vi "Project-overflow.vi"() -> ()   [LabVIEW 2016]
uses:
  <vilib>/DAQmx/read.llb/DAQmx Read (Digital Bool 1Line 1Point).vi
  <vilib>/DAQmx/write.llb/DAQmx Write (Digital Bool 1Line 1Point).vi
  <vilib>/DAQmx/create/channels.llb/DAQmx Create Channel (DO-Digital Output).vi
  <vilib>/DAQmx/create/channels.llb/DAQmx Create Channel (DI-Digital Input).vi
  <vilib>/DAQmx/miscellaneous.llb/DAQmx Fill In Error Info.vi
  <vilib>/ptbypt/NI_PtbyPt.lvlib
panel:
  out "Use R3":bool
  out "Register Bit 3":bool
  out "Laser Sensor":bool
  out "Use R2":bool
  out "Use R1":bool
  out "Register Bit 1":bool
  out "Register Bit 2":bool
  out "Output Queue Counter":dbl
  out "Rejection Pusher":bool
  out "Metal Sensor 2":bool
  out "Inductive Sensor":bool
  out "Complete or not":bool
  out "Plastic In Queue":dbl
  out "Hopper":bool
  out "Pusher":bool=TRUE
  out "Plastic or not":bool
  out "Belt 2":bool=TRUE
  out "Belt 1":bool=TRUE
  out "Stoped":bool=TRUE
  out "Started":bool=TRUE
  in  "PAUSE":bool
  in  "OFF":bool
  in  "ON":bool
  out "Rejected Pieces":dbl
  out "Completed Pieces":dbl
  out "Don't Push?":bool
  in  "Emergency Stop":bool
  out "Is there anything there?":bool
  # "Main Control"
  # "Sorting Station"
  # "QA Sorting Station"
  # "QA Sorting Register Value"
  # "Result Counter"
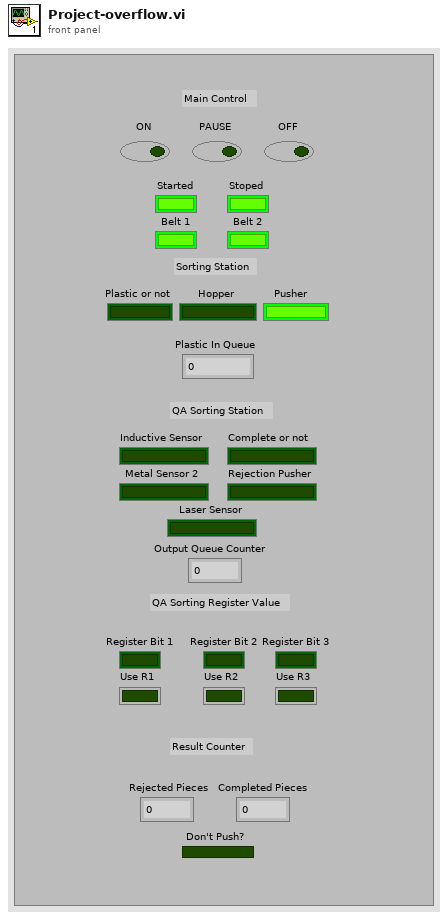
[diagram p1: front panel]
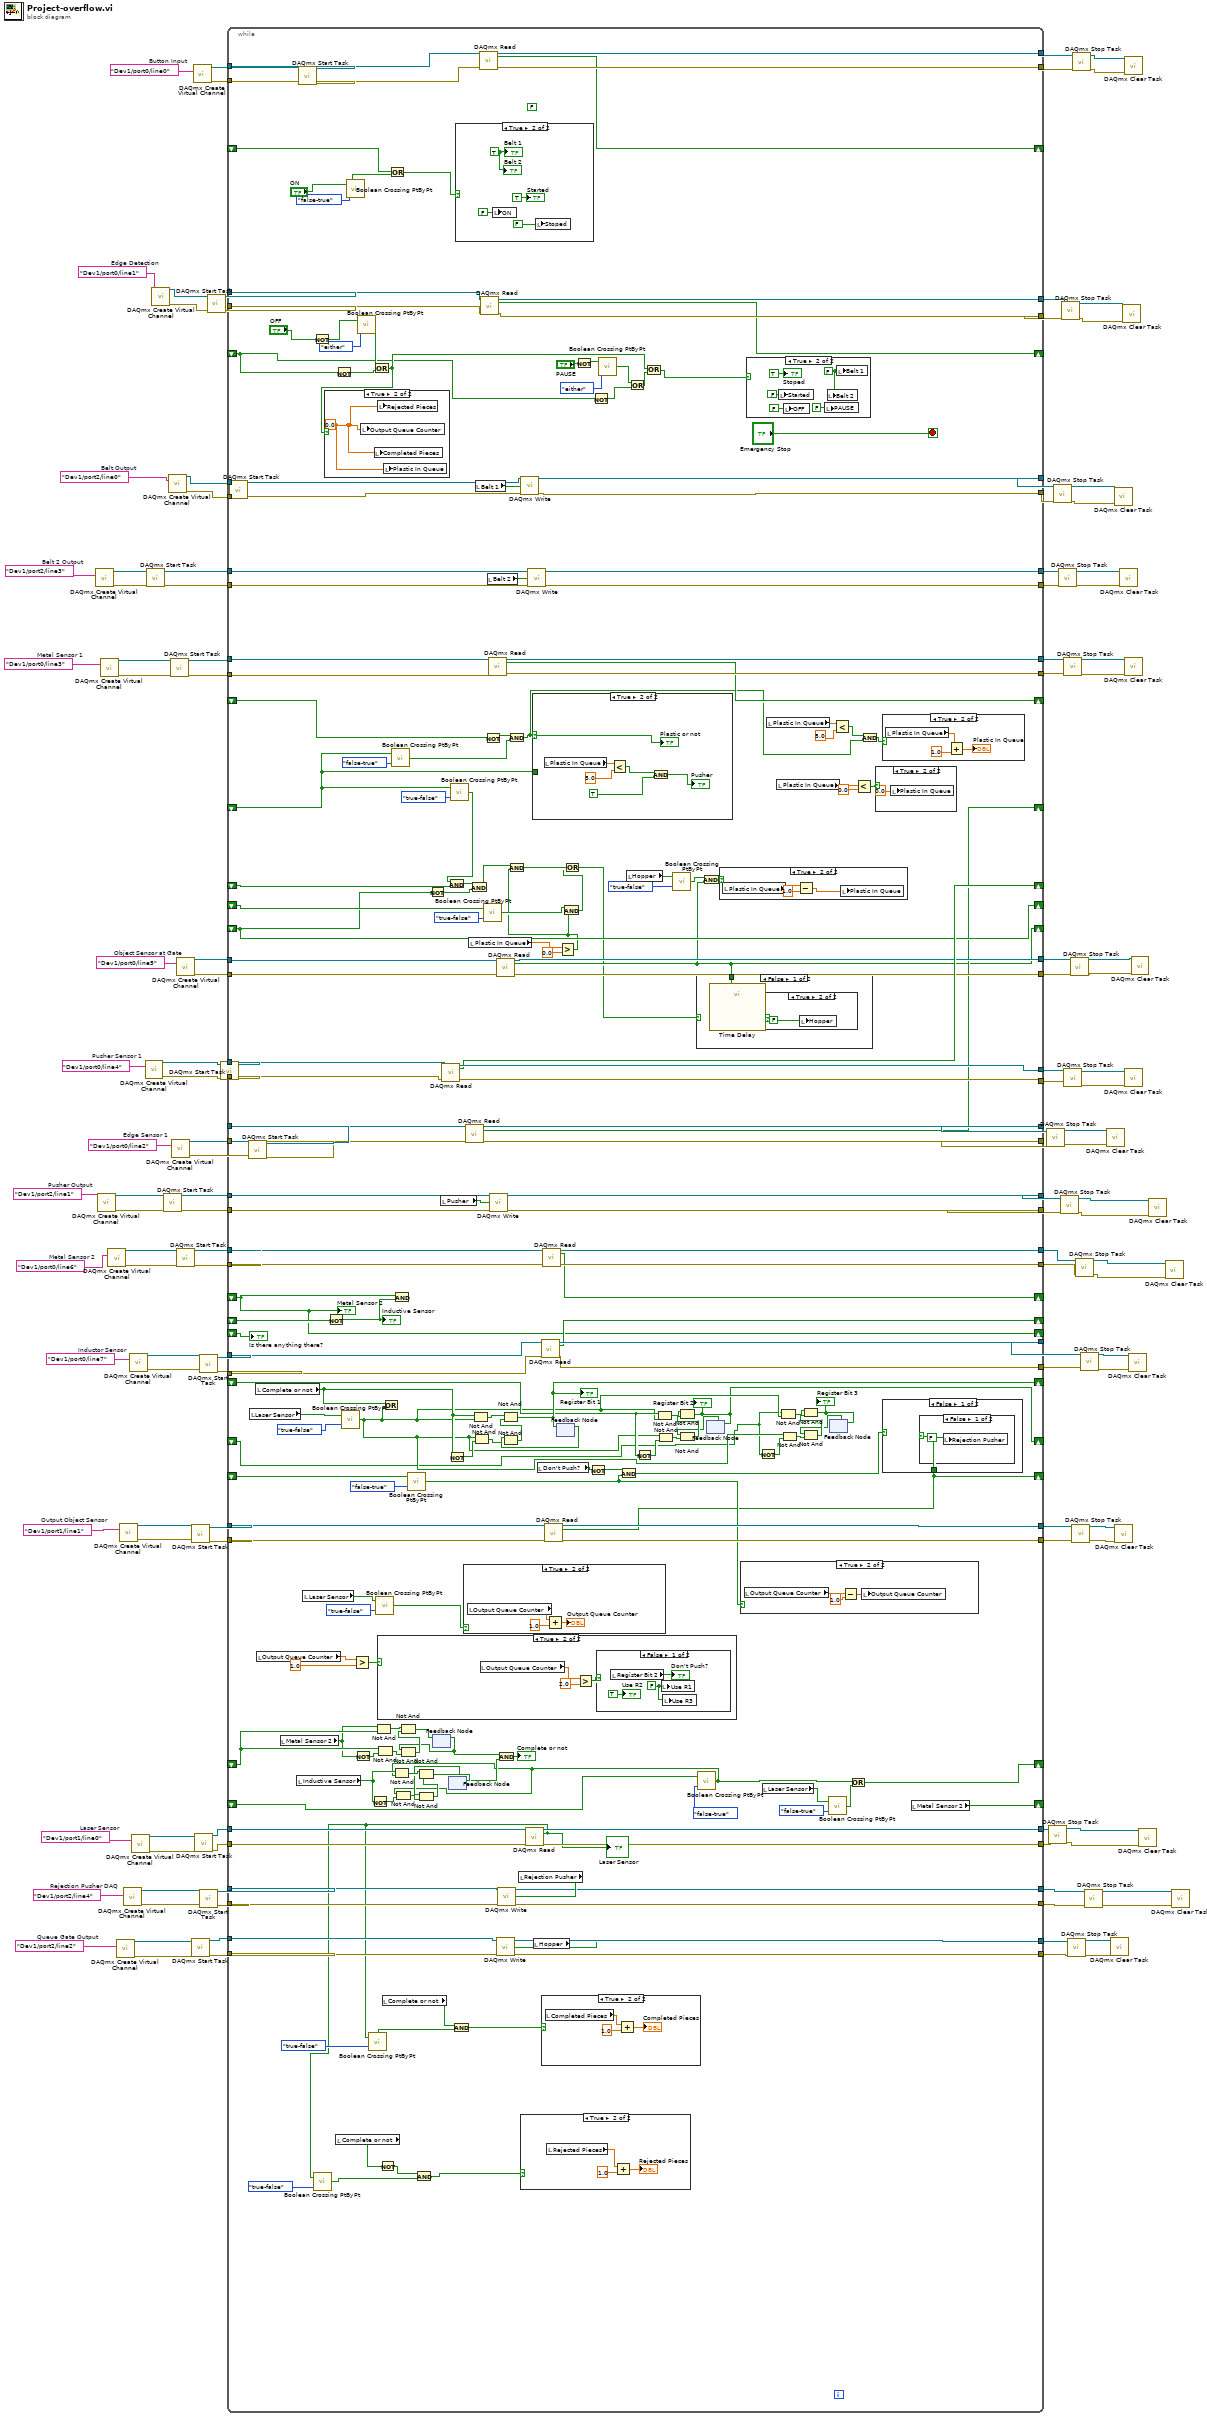
[diagram p0: block diagram]
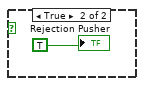
[diagram p3: hidden frame]
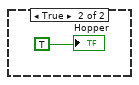
[diagram p5: hidden frame]
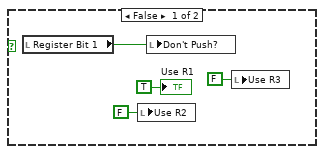
[diagram p12: hidden frame]
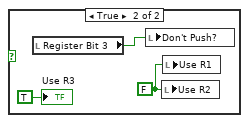
[diagram p13: hidden frame]
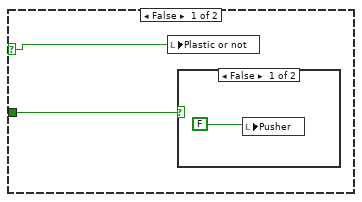
[diagram p16: hidden frame]
diagram:
  w5 = tag "Dev1/port0/line5"  # Object Sensor at Gate
  w12 = tag "Dev1/port1/line0"  # Laser Sensor
  w25 = tag "Dev1/port0/line7"  # Inductor Sensor
  w28 = tag "Dev1/port1/line1"  # Output Object Sensor
  w43 = tag "Dev1/port0/line6"  # Metal Sensor 2
  w46 = tag "Dev1/port2/line4"  # Rejection Pusher DAQ
  w57 = tag "Dev1/port2/line2"  # Queue Gate Output
  w64 = tag "Dev1/port2/line3"  # Belt 2 Output
  w75 = tag "Dev1/port0/line4"  # Pusher Sensor 1
  w84 = tag "Dev1/port0/line2"  # Edge Sensor 1
  w89 = tag "Dev1/port2/line1"  # Pusher Output
  w90 = tag "Dev1/port0/line1"  # Edge Detection
  w91 = tag "Dev1/port0/line0"  # Button Input
  w92 = tag "Dev1/port0/line3"  # Metal Sensor 1
  w93 = tag "Dev1/port2/line0"  # Belt Output
  n1 = call-poly <vilib>:"DAQmx Create Virtual Channel.vi"("lines"=w64) -> ("task out"=w66:refnum<k21>, "error out"=w65:errorcluster)  [unwired: 13 in]
  n2 = call-poly <vilib>:"DAQmx Create Virtual Channel.vi"("lines"=w89) -> ("task out"=w101:refnum<k21>, "error out"=w100:errorcluster)  [unwired: 13 in]
  n3 = call-poly <vilib>:"DAQmx Create Virtual Channel.vi"("lines"=w92) -> ("task out"=w109:refnum<k21>, "error out"=w108:errorcluster)  [unwired: 13 in]
  n4 = call-poly <vilib>:"DAQmx Create Virtual Channel.vi"("lines"=w43) -> ("task out"=w45:refnum<k21>, "error out"=w44:errorcluster)  [unwired: 13 in]
  n5 = call-poly <vilib>:"DAQmx Create Virtual Channel.vi"("lines"=w57) -> ("task out"=w59:refnum<k21>, "error out"=w58:errorcluster)  [unwired: 13 in]
  n6 = call-poly <vilib>:"DAQmx Create Virtual Channel.vi"("lines"=w28) -> ("task out"=w30:refnum<k21>, "error out"=w29:errorcluster)  [unwired: 13 in]
  n7 = call-poly <vilib>:"DAQmx Create Virtual Channel.vi"("lines"=w46) -> ("task out"=w48:refnum<k21>, "error out"=w47:errorcluster)  [unwired: 13 in]
  n8 = call-poly <vilib>:"DAQmx Create Virtual Channel.vi"("lines"=w25) -> ("task out"=w27:refnum<k21>, "error out"=w26:errorcluster)  [unwired: 13 in]
  n9 = call-poly <vilib>:"DAQmx Create Virtual Channel.vi"("lines"=w12) -> ("task out"=w14:refnum<k21>, "error out"=w13:errorcluster)  [unwired: 13 in]
  n10 = call-poly <vilib>:"DAQmx Create Virtual Channel.vi"("lines"=w75) -> ("task out"=w77:refnum<k21>, "error out"=w76:errorcluster)  [unwired: 13 in]
  n11 = call <vilib>:"DAQmx Start Task.vi"("task/channels in"=w66, "error in"=w65) -> ("task out"=w63:refnum<k21>, "error out"=w62:errorcluster)  [unwired: 12 in]
  n12 = call-poly <vilib>:"DAQmx Create Virtual Channel.vi"("lines"=w90) -> ("task out"=w125:refnum<k21>, "error out"=w124:errorcluster)  [unwired: 13 in]
  n13 = call <vilib>:"DAQmx Start Task.vi"("task/channels in"=w101, "error in"=w100) -> ("task out"=w95:refnum<k21>, "error out"=w94:errorcluster)  [unwired: 12 in]
  n14 = call-poly <vilib>:"DAQmx Create Virtual Channel.vi"("lines"=w93) -> ("task out"=w113:refnum<k21>, "error out"=w112:errorcluster)  [unwired: 13 in]
  n15 = call <vilib>:"DAQmx Start Task.vi"("task/channels in"=w109, "error in"=w108) -> ("task out"=w107:refnum<k21>, "error out"=w106:errorcluster)  [unwired: 12 in]
  n16 = call-poly <vilib>:"DAQmx Create Virtual Channel.vi"("lines"=w84) -> ("task out"=w86:refnum<k21>, "error out"=w85:errorcluster)  [unwired: 13 in]
  n17 = call <vilib>:"DAQmx Start Task.vi"("task/channels in"=w45, "error in"=w44) -> ("task out"=w40:refnum<k21>, "error out"=w39:errorcluster)  [unwired: 12 in]
  n18 = call-poly <vilib>:"DAQmx Create Virtual Channel.vi"("lines"=w5) -> ("task out"=w4:refnum<k21>, "error out"=w3:errorcluster)  [unwired: 13 in]
  n19 = call <vilib>:"DAQmx Start Task.vi"("task/channels in"=w30, "error in"=w29) -> ("task out"=w24:refnum<k21>, "error out"=w23:errorcluster)  [unwired: 12 in]
  n20 = call <vilib>:"DAQmx Start Task.vi"("task/channels in"=w59, "error in"=w58) -> ("task out"=w56:refnum<k21>, "error out"=w55:errorcluster)  [unwired: 12 in]
  n21 = call-poly <vilib>:"DAQmx Create Virtual Channel.vi"("lines"=w91) -> ("task out"=w133:refnum<k21>, "error out"=w132:errorcluster)  [unwired: 13 in]
  n22 = call <vilib>:"DAQmx Start Task.vi"("task/channels in"=w14, "error in"=w13) -> ("task out"=w11:refnum<k21>, "error out"=w8:errorcluster)  [unwired: 12 in]
  n23 = call <vilib>:"DAQmx Start Task.vi"("task/channels in"=w27, "error in"=w26) -> ("task out"=w22:refnum<k21>, "error out"=w21:errorcluster)  [unwired: 12 in]
  n24 = call <vilib>:"DAQmx Start Task.vi"("task/channels in"=w48, "error in"=w47) -> ("task out"=w38:refnum<k21>, "error out"=w37:errorcluster)  [unwired: 12 in]
  n25 = call <vilib>:"DAQmx Start Task.vi"("task/channels in"=w125, "error in"=w124) -> ("task out"=w122:refnum<k21>, "error out"=w123:errorcluster)  [unwired: 12 in]
  n26 = call <vilib>:"DAQmx Start Task.vi"("task/channels in"=w77, "error in"=w76) -> ("task out"=w74:refnum<k21>, "error out"=w73:errorcluster)  [unwired: 12 in]
  n27 = call <vilib>:"DAQmx Start Task.vi"("task/channels in"=w113, "error in"=w112) -> ("task out"=w111:refnum<k21>, "error out"=w110:errorcluster)  [unwired: 12 in]
  n28 = call <vilib>:"DAQmx Start Task.vi"("task/channels in"=w86, "error in"=w85) -> ("task out"=w83:refnum<k21>, "error out"=w82:errorcluster)  [unwired: 12 in]
  n29 = call <vilib>:"DAQmx Start Task.vi"("task/channels in"=w133, "error in"=w132) -> ("task out"=w131:refnum<k21>, "error out"=w130:errorcluster)  [unwired: 12 in]
  n30 = while {
    tunnel: w131 -> [w334]
    tunnel: w130 -> [w333]
    tunnel: [w332] -> w129
    tunnel: [w331] -> w128
    shift-right: [w329] -> _
    shift-left: _ -> [w263]
    tunnel: w123 -> [w328]
    tunnel: w122 -> [w327]
    tunnel: [w326] -> w121
    tunnel: [w325] -> w118
    shift-right: [w324] -> _
    shift-left: _ -> [w203]
    tunnel: [w323] -> w115
    tunnel: [w320] -> w114
    tunnel: w111 -> [w322]
    tunnel: w110 -> [w321]
    tunnel: w107 -> [w318]
    tunnel: w106 -> [w317]
    tunnel: [w316] -> w103
    tunnel: [w315] -> w102
    shift-right: [w178] -> _
    shift-left: _ -> [w177]
    tunnel: [w313] -> w97
    tunnel: [w312] -> w96
    tunnel: w95 -> [w311]
    tunnel: w94 -> [w310]
    tunnel: w83 -> [w309]
    tunnel: w82 -> [w308]
    tunnel: [w307] -> w81
    tunnel: [w306] -> w80
    shift-right: [w180] -> _
    shift-left: _ -> [w173]
    tunnel: w74 -> [w304]
    tunnel: w73 -> [w303]
    tunnel: [w302] -> w72
    tunnel: [w301] -> w71
    tunnel: [w298] -> w68
    tunnel: [w297] -> w67
    tunnel: w63 -> [w296]
    tunnel: w62 -> [w295]
    tunnel: w56 -> [w294]
    tunnel: w55 -> [w293]
    tunnel: [w292] -> w54
    tunnel: [w291] -> w53
    shift-right: [w289] -> _
    shift-left: _ -> [w288]
    tunnel: [w284] -> w42
    tunnel: [w283] -> w41
    tunnel: w40 -> [w282]
    tunnel: w39 -> [w281]
    tunnel: w38 -> [w280]
    tunnel: w37 -> [w279]
    tunnel: [w278] -> w36
    tunnel: [w277] -> w35
    shift-right: [w276] -> _
    shift-left: _ -> [w230]
    tunnel: w24 -> [w275]
    tunnel: w23 -> [w274]
    tunnel: w22 -> [w273]
    tunnel: w21 -> [w272]
    tunnel: [w271] -> w20
    tunnel: [w270] -> w19
    tunnel: [w269] -> w18
    tunnel: [w268] -> w17
    shift-right: [w181] -> _
    shift-left: _ -> [w251]
    shift-right: [w267] -> _
    shift-left: _ -> [w266]
    shift-right: [w230] -> _
    shift-left: _ -> [w253]
    tunnel: w11 -> [w249]
    tunnel: [w248] -> w10
    tunnel: [w247] -> w9
    tunnel: w8 -> [w246]
    shift-right: [w232] -> _
    shift-left: _ -> [w231]
    tunnel: w4 -> [w202]
    tunnel: w3 -> [w201]
    tunnel: [w200] -> w2
    tunnel: [w199] -> w1
    shift-right: [w175] -> _
    shift-left: _ -> [w194]
    shift-right: [w194] -> _
    shift-left: _ -> [w197]
    shift-right: [w154] -> _
    shift-left: _ -> [w166]
    shift-right: [w137] -> _
    shift-left: _ -> [w136]
    shift-right: [w135] -> _
    shift-left: _ -> [w134]
    stop <- "Emergency Stop" stop-if-true
    (unwired) FALSE ("Boolean")
    n31 = local read "Laser Sensor"() -> (w254:bool)
    n32 = local read "Complete or not"() -> (w229:bool)
    n33 = local read "Output Queue Counter"() -> (w239:dbl)
    n34 = local read "Metal Sensor 2"() -> (w165:bool)
    n35 = local read "Inductive Sensor"() -> (w159:bool)
    n36 = local read "Laser Sensor"() -> (w243:bool)
    n37 = Not(x="OFF") -> (.not. x?=w225:bool)
    n38 = Not(x=w266) -> (.not. x?=w261:bool)
    "Inductive Sensor" <- w261
    n39 = Not(x=w203) -> (.not. x?=w262:bool)
    n40 = local read "Complete or not"() -> (w212:bool)
    n41 = call <vilib>:"Boolean Crossing PtByPt.vi"("direction"=enum16{"either", "false-true", "true-false"}."true-false", "input"=w254) -> ("crossing"=w144:bool)  [unwired: 1 in]
    n42 = call <vilib>:"Boolean Crossing PtByPt.vi"("direction"=enum16{"either", "false-true", "true-false"}."false-true", "input"="ON") -> ("crossing"=w228:bool)  [unwired: 1 in]
    n43 = Greater?(x=w239, y=1.0) -> (0:w238:bool)
    n44 = Not(x=w165) -> (.not. x?=w169:bool)
    n45 = call <vilib>:"Boolean Crossing PtByPt.vi"("direction"=enum16{"either", "false-true", "true-false"}."either", "input"=w225) -> ("crossing"=w226:bool)  [unwired: 1 in]
    n46 = Not(x=w159) -> (.not. x?=w161:bool)
    n47 = Or(x=w226, y=w262) -> (x .or. y?=w204:bool)
    n48 = case shown="True" w204 {
      frame False {
      }
      frame True {
        w348 = 0.0 ("Completed Piece")
        n49 = local write "Output Queue Counter"(w348) -> ()
        n50 = local write "Completed Pieces"(w348) -> ()
        n51 = local write "Rejected Pieces"(w348) -> ()
        n52 = local write "Plastic In Queue"(w348) -> ()
      }
    }
    n53 = Not And(1:w166, 2:w165) -> (0:w170:bool)
    n54 = call <vilib>:"Boolean Crossing PtByPt.vi"("direction"=enum16{"either", "false-true", "true-false"}."true-false", "input"=w243) -> ("crossing"=w244:bool)  [unwired: 1 in]
    n55 = Not And(1:w169, 2:w166) -> (0:w171:bool)
    n56 = case shown="True" w238 {
      frame False {
        n57 = local read "Register Bit 1"() -> (w358:bool)
        n58 = local write "Use R2"(FALSE ("Use R2")) -> ()
        n59 = local write "Don't Push?"(w358) -> ()
        n60 = local write "Use R3"(FALSE ("Use R3")) -> ()
        "Use R1" <- TRUE ("Use R1")
      }
      frame True {
        n61 = local read "Output Queue Counter"() -> (w361:dbl)
        n62 = Greater?(x=w361, y=2.0) -> (0:w359:bool)
        n63 = case shown="False" w359 {
          frame False {
            w362 = FALSE ("Use R1")
            n64 = local read "Register Bit 2"() -> (→"Don't Push?":bool)
            n65 = local write "Use R1"(w362) -> ()
            n66 = local write "Use R3"(w362) -> ()
            "Use R2" <- TRUE ("Use R2")
          }
          frame True {
            w365 = FALSE ("Use R2")
            n67 = local read "Register Bit 3"() -> (w366:bool)
            n68 = local write "Don't Push?"(w366) -> ()
            n69 = local write "Use R2"(w365) -> ()
            n70 = local write "Use R1"(w365) -> ()
            "Use R3" <- TRUE ("Use R3")
          }
        }
      }
    }
    n71 = Not(x=w212) -> (.not. x?=w213:bool)
    n72 = Or(x=w229, y=w144) -> ()  [unwired: 1 out]
    n73 = local read "Complete or not"() -> (w219:bool)
    n74 = Or(x=w263, y=w228) -> (x .or. y?=w264:bool)
    n75 = call <vilib>:"Boolean Crossing PtByPt.vi"("direction"=enum16{"either", "false-true", "true-false"}."false-true", "input"=w173) -> ("crossing"=w290:bool)  [unwired: 1 in]
    n76 = And(x=w230, y=w261) -> ()  [unwired: 1 out]
    n77 = call <vilib>:"Boolean Crossing PtByPt.vi"("direction"=enum16{"either", "false-true", "true-false"}."false-true", "input"=w251) -> ("crossing"=w241:bool)  [unwired: 1 in]
    n78 = Not(x=w194) -> (.not. x?=w195:bool)
    n79 = feedback #1() -> (w158:bool)  [unwired: 1 in]
    n80 = Not And(1:w171, 2:w158) -> (0:w172:bool)
    n81 = Not And(1:w172, 2:w170) -> (0:w168:bool)
    n82 = feedback-in #1(w168) -> ()
    n83 = local read "Pusher"() -> (w314:bool)
    n84 = call-poly <vilib>:"DAQmx Read.vi"("task/channels in"=w304, "error in"=w303) -> ("task out"=w301:refnum<k21>, "data"=w289:bool, "error out"=w302:errorcluster)  [unwired: 11 in]
    n85 = Not(x=w229) -> (.not. x?=w256:bool)
    n86 = feedback #2() -> (w157:bool)  [unwired: 1 in]
    n87 = call <vilib>:"Boolean Crossing PtByPt.vi"("direction"=enum16{"either", "false-true", "true-false"}."true-false", "input"=w173) -> ("crossing"=w286:bool)  [unwired: 1 in]
    n88 = And(x=w286, y=w288) -> (x .and. y?=w196:bool)
    n89 = case shown="True" w264 {
      frame False {
      }
      frame True {
        w389 = TRUE
        n90 = local write "ON"(FALSE ("ON")) -> ()
        n91 = local write "Stoped"(FALSE) -> ()
        "Started" <- TRUE ("Boolean")
        "Belt 1" <- w389
        "Belt 2" <- w389
      }
    }
    n92 = case shown="True" w244 {
      frame False {
      }
      frame True {
        n93 = local read "Output Queue Counter"() -> (w371:dbl)
        n94 = Add(x=w371, y=1.0) -> (x+y=→"Output Queue Counter":dbl)
      }
    }
    n95 = call-poly <vilib>:"DAQmx Read.vi"("task/channels in"=w309, "error in"=w308) -> ("task out"=w306:refnum<k21>, "data"=w180:bool, "error out"=w307:errorcluster)  [unwired: 11 in]
    n96 = local read "Plastic In Queue"() -> (w193:dbl)
    n97 = And(x=w196, y=w195) -> (x .and. y?=w189:bool)
    n98 = Not And(1:w144, 2:w229) -> (0:w257:bool)
    n99 = Not And(1:w256, 2:w144) -> (0:w258:bool)
    n100 = local read "Belt 1"() -> (w319:bool)
    n101 = call-poly <vilib>:"DAQmx Read.vi"("task/channels in"=w334, "error in"=w333) -> ("task out"=w332:refnum<k21>, "data"=w329:bool, "error out"=w331:errorcluster)  [unwired: 11 in]
    n102 = call-poly <vilib>:"DAQmx Read.vi"("task/channels in"=w327, "error in"=w328) -> ("task out"=w326:refnum<k21>, "data"=w324:bool, "error out"=w325:errorcluster)  [unwired: 11 in]
    n103 = call <vilib>:"Boolean Crossing PtByPt.vi"("direction"=enum16{"either", "false-true", "true-false"}."true-false", "input"=w197) -> ("crossing"=w191:bool)  [unwired: 1 in]
    n104 = Not(x=w177) -> (.not. x?=w305:bool)
    n105 = local read "Belt 2"() -> (w299:bool)
    n106 = call-poly <vilib>:"DAQmx Read.vi"("task/channels in"=w318, "error in"=w317) -> ("task out"=w316:refnum<k21>, "data"=w178:bool, "error out"=w315:errorcluster)  [unwired: 11 in]
    n107 = call-poly <vilib>:"DAQmx Write.vi"("task/channels in"=w311, "data"=w314, "error in"=w310) -> ("task out"=w313:refnum<k21>, "error out"=w312:errorcluster)  [unwired: 10 in, 1 out]
    n108 = call-poly <vilib>:"DAQmx Read.vi"("task/channels in"=w202, "error in"=w201) -> ("task out"=w200:refnum<k21>, "data"=w175:bool, "error out"=w199:errorcluster)  [unwired: 11 in]
    n109 = And(x=w158, y=w157) -> (x .and. y?=→"Complete or not":bool)
    n110 = And(x=w305, y=w290) -> (x .and. y?=w139:bool)
    n111 = local read "Rejection Pusher"() -> (w285:bool)
    n112 = call-poly <vilib>:"DAQmx Write.vi"("task/channels in"=w280, "data"=w285, "error in"=w279) -> ("task out"=w278:refnum<k21>, "error out"=w277:errorcluster)  [unwired: 10 in, 1 out]
    n113 = call-poly <vilib>:"DAQmx Write.vi"("task/channels in"=w322, "data"=w319, "error in"=w321) -> ("task out"=w323:refnum<k21>, "error out"=w320:errorcluster)  [unwired: 10 in, 1 out]
    n114 = call-poly <vilib>:"DAQmx Read.vi"("task/channels in"=w249, "error in"=w246) -> ("task out"=w248:refnum<k21>, "data"=w216:bool, "error out"=w247:errorcluster)  [unwired: 11 in]
    "Laser Sensor" <- w216
    n115 = call <vilib>:"Boolean Crossing PtByPt.vi"("direction"=enum16{"either", "false-true", "true-false"}."true-false", "input"=w216) -> ("crossing"=w214:bool)  [unwired: 1 in]
    n116 = call <vilib>:"Boolean Crossing PtByPt.vi"("direction"=enum16{"either", "false-true", "true-false"}."true-false", "input"=w216) -> ("crossing"=w218:bool)  [unwired: 1 in]
    n117 = And(x=w213, y=w214) -> (x .and. y?=w215:bool)
    n118 = And(x=w219, y=w218) -> (x .and. y?=w217:bool)
    n119 = case shown="True" w215 {
      frame False {
      }
      frame True {
        n120 = local read "Rejected Pieces"() -> (w350:dbl)
        n121 = Add(x=w350, y=1.0) -> (x+y=→"Rejected Pieces":dbl)
      }
    }
    n122 = call-poly <vilib>:"DAQmx Write.vi"("task/channels in"=w296, "data"=w299, "error in"=w295) -> ("task out"=w298:refnum<k21>, "error out"=w297:errorcluster)  [unwired: 10 in, 1 out]
    n123 = case shown="True" w139 {
      selector: w139 -> [w375 w382]
      tunnel: w173 -> [w374 _]
      frame False {
        n124 = local write "Plastic or not"(w375) -> ()
        n125 = case shown="False" w374 {
          frame False {
            n126 = local write "Pusher"(FALSE) -> ()
          }
          frame True {
          }
        }
      }
      frame True {
        n127 = local read "Plastic In Queue"() -> (w380:dbl)
        n128 = Less?(x=w380, y=5.0) -> (x < y?=w379:bool)
        n129 = And(x=w379, y=TRUE) -> (x .and. y?=→"Pusher":bool)
        "Plastic or not" <- w382
      }
    }
    n130 = local read "Hopper"() -> (w265:bool)
    n131 = call-poly <vilib>:"DAQmx Write.vi"("task/channels in"=w294, "data"=w265, "error in"=w293) -> ("task out"=w292:refnum<k21>, "error out"=w291:errorcluster)  [unwired: 10 in, 1 out]
    n132 = local read "Don't Push?"() -> (w245:bool)
    n133 = call-poly <vilib>:"DAQmx Read.vi"("task/channels in"=w273, "error in"=w272) -> ("task out"=w268:refnum<k21>, "data"=w267:bool, "error out"=w269:errorcluster)  [unwired: 11 in]
    n134 = case shown="True" w217 {
      frame False {
      }
      frame True {
        n135 = local read "Completed Pieces"() -> (w352:dbl)
        n136 = Add(x=w352, y=1.0) -> (x+y=→"Completed Pieces":dbl)
      }
    }
    n137 = call-poly <vilib>:"DAQmx Read.vi"("task/channels in"=w282, "error in"=w281) -> ("task out"=w284:refnum<k21>, "data"=w276:bool, "error out"=w283:errorcluster)  [unwired: 11 in]
    n138 = call-poly <vilib>:"DAQmx Read.vi"("task/channels in"=w275, "error in"=w274) -> ("task out"=w271:refnum<k21>, "data"=w181:bool, "error out"=w270:errorcluster)  [unwired: 11 in]
    n139 = feedback #3() -> (w259:bool)  [unwired: 1 in]
    n140 = Not And(1:w258, 2:w259) -> (0:w260:bool)
    n141 = Not And(1:w260, 2:w257) -> (0:w232:bool)
    "Register Bit 1" <- w232
    n142 = feedback-in #3(w232) -> ()
    n143 = Greater?(x=w193, y=0.0) -> (0:w188:bool)
    n144 = And(x=w189, y=w188) -> (x .and. y?=w184:bool)
    n145 = And(x=w191, y=w188) -> (x .and. y?=w183:bool)
    n146 = Or(x=w184, y=w183) -> (x .or. y?=w143:bool)
    n147 = Not(x="PAUSE") -> (.not. x?=w209:bool)
    n148 = Not(x=w245) -> (.not. x?=w252:bool)
    n149 = Not(x=w203) -> (.not. x?=w211:bool)
    n150 = call <vilib>:"Boolean Crossing PtByPt.vi"("direction"=enum16{"either", "false-true", "true-false"}."either", "input"=w209) -> ("crossing"=w210:bool)  [unwired: 1 in]
    n151 = And(x=w252, y=w241) -> (x .and. y?=w182:bool)
    n152 = local read "Hopper"() -> (w179:bool)
    n153 = Or(x=w210, y=w211) -> (x .or. y?=w205:bool)
    n154 = Not(x=w231) -> (.not. x?=w233:bool)
    n155 = Or(x=w204, y=w205) -> (x .or. y?=w206:bool)
    n156 = Not And(1:w144, 2:w231) -> (0:w234:bool)
    n157 = Not And(1:w233, 2:w144) -> (0:w235:bool)
    n158 = call <vilib>:"Boolean Crossing PtByPt.vi"("direction"=enum16{"either", "false-true", "true-false"}."true-false", "input"=w179) -> ("crossing"=w176:bool)  [unwired: 1 in]
    n159 = case shown="False" w143 {
      tunnel: w175 -> [w338 _]
      frame False {
        n160 = call "Time Delay"() -> ()  [unwired: 11 in, 1 out]
        n161 = case shown="True" w338 {
          frame False {
          }
          frame True {
            n162 = local write "Hopper"(FALSE) -> ()
          }
        }
      }
      frame True {
        "Hopper" <- TRUE
      }
    }
    n163 = call <vilib>:"Boolean Crossing PtByPt.vi"("direction"=enum16{"either", "false-true", "true-false"}."false-true", "input"=w136) -> ("crossing"=w155:bool)  [unwired: 1 in]
    n164 = Not And(1:w155, 2:w159) -> (0:w162:bool)
    n165 = Not And(1:w161, 2:w155) -> (0:w163:bool)
    n166 = Not And(1:w163, 2:w157) -> (0:w164:bool)
    n167 = Not And(1:w164, 2:w162) -> (0:w160:bool)
    n168 = feedback-in #2(w160) -> ()
    n169 = And(x=w176, y=w175) -> (x .and. y?=w174:bool)
    n170 = feedback #4() -> (w236:bool)  [unwired: 1 in]
    n171 = Not And(1:w235, 2:w236) -> (0:w237:bool)
    n172 = Not And(1:w237, 2:w234) -> (0:w135:bool)
    "Register Bit 2" <- w135
    n173 = feedback-in #4(w135) -> ()
    n174 = case shown="True" w174 {
      frame False {
      }
      frame True {
        n175 = local read "Plastic In Queue"() -> (w343:dbl)
        n176 = Subtract(x=w343, y=1.0) -> (x-y=w344:dbl)
        n177 = local write "Plastic In Queue"(w344) -> ()
      }
    }
    n178 = case shown="True" w241 {
      frame False {
      }
      frame True {
        n179 = local read "Output Queue Counter"() -> (w370:dbl)
        n180 = Subtract(x=w370, y=1.0) -> (x-y=w368:dbl)
        n181 = local write "Output Queue Counter"(w368) -> ()
      }
    }
    n182 = case shown="True" w206 {
      frame False {
      }
      frame True {
        w385 = FALSE
        n183 = local write "Started"(FALSE ("Stop")) -> ()
        n184 = local write "OFF"(FALSE ("OFF")) -> ()
        n185 = local write "PAUSE"(FALSE ("Pause")) -> ()
        n186 = local write "Belt 2"(w385) -> ()
        n187 = local write "Belt 1"(w385) -> ()
        "Stoped" <- TRUE
      }
    }
    n188 = Not(x=w134) -> (.not. x?=w146:bool)
    n189 = local read "Laser Sensor"() -> (w152:bool)
    n190 = local read "Plastic In Queue"() -> (w141:dbl)
    n191 = local read "Plastic In Queue"() -> (w187:dbl)
    n192 = Not And(1:w144, 2:w134) -> (0:w147:bool)
    n193 = Not And(1:w146, 2:w144) -> (0:w148:bool)
    n194 = call <vilib>:"Boolean Crossing PtByPt.vi"("direction"=enum16{"either", "false-true", "true-false"}."false-true", "input"=w152) -> ("crossing"=w151:bool)  [unwired: 1 in]
    n195 = feedback #5() -> (w149:bool)  [unwired: 1 in]
    n196 = Not And(1:w148, 2:w149) -> (0:w150:bool)
    n197 = Not And(1:w150, 2:w147) -> (0:w145:bool)
    "Register Bit 3" <- w145
    n198 = feedback-in #5(w145) -> ()
    n199 = Less?(x=w141, y=5.0) -> (x < y?=w142:bool)
    n200 = Or(x=w155, y=w151) -> (x .or. y?=w154:bool)
    n201 = Less?(x=w187, y=0.0) -> (x < y?=w185:bool)
    n202 = And(x=w142, y=w139) -> (x .and. y?=w138:bool)
    n203 = case shown="True" w185 {
      frame False {
      }
      frame True {
        n204 = local write "Plastic In Queue"(0.0 ("Plastic In Queue")) -> ()
      }
    }
    n205 = case shown="True" w138 {
      frame False {
      }
      frame True {
        n206 = local read "Plastic In Queue"() -> (w345:dbl)
        n207 = Add(x=w345, y=1.0) -> (x+y=→"Plastic In Queue":dbl)
      }
    }
    n208 = case shown="False" w182 {
      tunnel: w181 -> [w335 _]
      frame False {
        n209 = case shown="False" w335 {
          frame False {
            n210 = local write "Rejection Pusher"(FALSE) -> ()
          }
          frame True {
          }
        }
      }
      frame True {
        "Rejection Pusher" <- TRUE
      }
    }
    n211 = local read "Metal Sensor 2"() -> (w137:bool)
    "Metal Sensor 2" <- w230
    "Is there anything there?" <- w253
  }
  n212 = call <vilib>:"DAQmx Stop Task.vi"("task/channels in"=w80, "error in"=w81) -> ("task out"=w88:refnum<k21>, "error out"=w87:errorcluster)  [unwired: 12 in]
  n213 = call <vilib>:"DAQmx Stop Task.vi"("task/channels in"=w10, "error in"=w9) -> ("task out"=w16:refnum<k21>, "error out"=w15:errorcluster)  [unwired: 12 in]
  n214 = call <vilib>:"DAQmx Stop Task.vi"("task/channels in"=w115, "error in"=w114) -> ("task out"=w117:refnum<k21>, "error out"=w116:errorcluster)  [unwired: 12 in]
  n215 = call <vilib>:"DAQmx Stop Task.vi"("task/channels in"=w68, "error in"=w67) -> ("task out"=w70:refnum<k21>, "error out"=w69:errorcluster)  [unwired: 12 in]
  n216 = call <vilib>:"DAQmx Stop Task.vi"("task/channels in"=w97, "error in"=w96) -> ("task out"=w99:refnum<k21>, "error out"=w98:errorcluster)  [unwired: 12 in]
  n217 = call <vilib>:"DAQmx Stop Task.vi"("task/channels in"=w121, "error in"=w118) -> ("task out"=w120:refnum<k21>, "error out"=w119:errorcluster)  [unwired: 12 in]
  n218 = call <vilib>:"DAQmx Stop Task.vi"("task/channels in"=w103, "error in"=w102) -> ("task out"=w105:refnum<k21>, "error out"=w104:errorcluster)  [unwired: 12 in]
  n219 = call <vilib>:"DAQmx Stop Task.vi"("task/channels in"=w71, "error in"=w72) -> ("task out"=w79:refnum<k21>, "error out"=w78:errorcluster)  [unwired: 12 in]
  n220 = call <vilib>:"DAQmx Stop Task.vi"("task/channels in"=w54, "error in"=w53) -> ("task out"=w61:refnum<k21>, "error out"=w60:errorcluster)  [unwired: 12 in]
  n221 = call <vilib>:"DAQmx Stop Task.vi"("task/channels in"=w2, "error in"=w1) -> ("task out"=w7:refnum<k21>, "error out"=w6:errorcluster)  [unwired: 12 in]
  n222 = call <vilib>:"DAQmx Stop Task.vi"("task/channels in"=w20, "error in"=w19) -> ("task out"=w34:refnum<k21>, "error out"=w33:errorcluster)  [unwired: 12 in]
  n223 = call <vilib>:"DAQmx Stop Task.vi"("task/channels in"=w129, "error in"=w128) -> ("task out"=w126:refnum<k21>, "error out"=w127:errorcluster)  [unwired: 12 in]
  n224 = call <vilib>:"DAQmx Stop Task.vi"("task/channels in"=w42, "error in"=w41) -> ("task out"=w50:refnum<k21>, "error out"=w49:errorcluster)  [unwired: 12 in]
  n225 = call <vilib>:"DAQmx Stop Task.vi"("task/channels in"=w17, "error in"=w18) -> ("task out"=w32:refnum<k21>, "error out"=w31:errorcluster)  [unwired: 12 in]
  n226 = call <vilib>:"DAQmx Stop Task.vi"("task/channels in"=w36, "error in"=w35) -> ("task out"=w52:refnum<k21>, "error out"=w51:errorcluster)  [unwired: 12 in]
  n227 = call <vilib>:"DAQmx Clear Task.vi"("task in"=w88, "error in"=w87) -> ()  [unwired: 13 in, 1 out]
  n228 = call <vilib>:"DAQmx Clear Task.vi"("task in"=w61, "error in"=w60) -> ()  [unwired: 13 in, 1 out]
  n229 = call <vilib>:"DAQmx Clear Task.vi"("task in"=w117, "error in"=w116) -> ()  [unwired: 13 in, 1 out]
  n230 = call <vilib>:"DAQmx Clear Task.vi"("task in"=w34, "error in"=w33) -> ()  [unwired: 13 in, 1 out]
  n231 = call <vilib>:"DAQmx Clear Task.vi"("task in"=w70, "error in"=w69) -> ()  [unwired: 13 in, 1 out]
  n232 = call <vilib>:"DAQmx Clear Task.vi"("task in"=w120, "error in"=w119) -> ()  [unwired: 13 in, 1 out]
  n233 = call <vilib>:"DAQmx Clear Task.vi"("task in"=w126, "error in"=w127) -> ()  [unwired: 13 in, 1 out]
  n234 = call <vilib>:"DAQmx Clear Task.vi"("task in"=w105, "error in"=w104) -> ()  [unwired: 13 in, 1 out]
  n235 = call <vilib>:"DAQmx Clear Task.vi"("task in"=w79, "error in"=w78) -> ()  [unwired: 13 in, 1 out]
  n236 = call <vilib>:"DAQmx Clear Task.vi"("task in"=w32, "error in"=w31) -> ()  [unwired: 13 in, 1 out]
  n237 = call <vilib>:"DAQmx Clear Task.vi"("task in"=w7, "error in"=w6) -> ()  [unwired: 13 in, 1 out]
  n238 = call <vilib>:"DAQmx Clear Task.vi"("task in"=w16, "error in"=w15) -> ()  [unwired: 13 in, 1 out]
  n239 = call <vilib>:"DAQmx Clear Task.vi"("task in"=w99, "error in"=w98) -> ()  [unwired: 13 in, 1 out]
  n240 = call <vilib>:"DAQmx Clear Task.vi"("task in"=w50, "error in"=w49) -> ()  [unwired: 13 in, 1 out]
  n241 = call <vilib>:"DAQmx Clear Task.vi"("task in"=w52, "error in"=w51) -> ()  [unwired: 13 in, 1 out]
